vi "Decodificador_7seg_SubVI.vi"(1 "A":bool, 2 "B":bool, 3 "C":bool, 4 "D":bool) -> (0 "DISPLAY":T1)   [LabVIEW 2016]
doc: "Esta SubVI nos entrega a la salida un cluster que nos representa un dato binario en display de 7 segmentos."
panel:
  out "Segmento B":bool
  out "Segmento C":bool
  out "Segmento D":bool
  out "Segmento E":bool
  out "Segmento F":bool
  out "Segmento G":bool
  out "Segmento A":bool
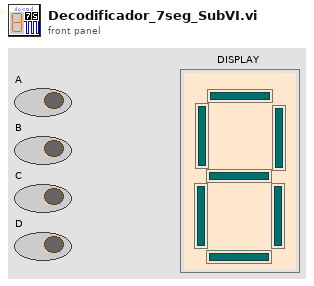
[diagram p1: front panel]
types:
  T1 = cluster{"SA":bool, "SB":bool, "SC":bool, "SD":bool, "SE":bool, "SF":bool, "SG":bool}
  T2 = cluster{bool, bool, bool, bool, bool, bool, bool}
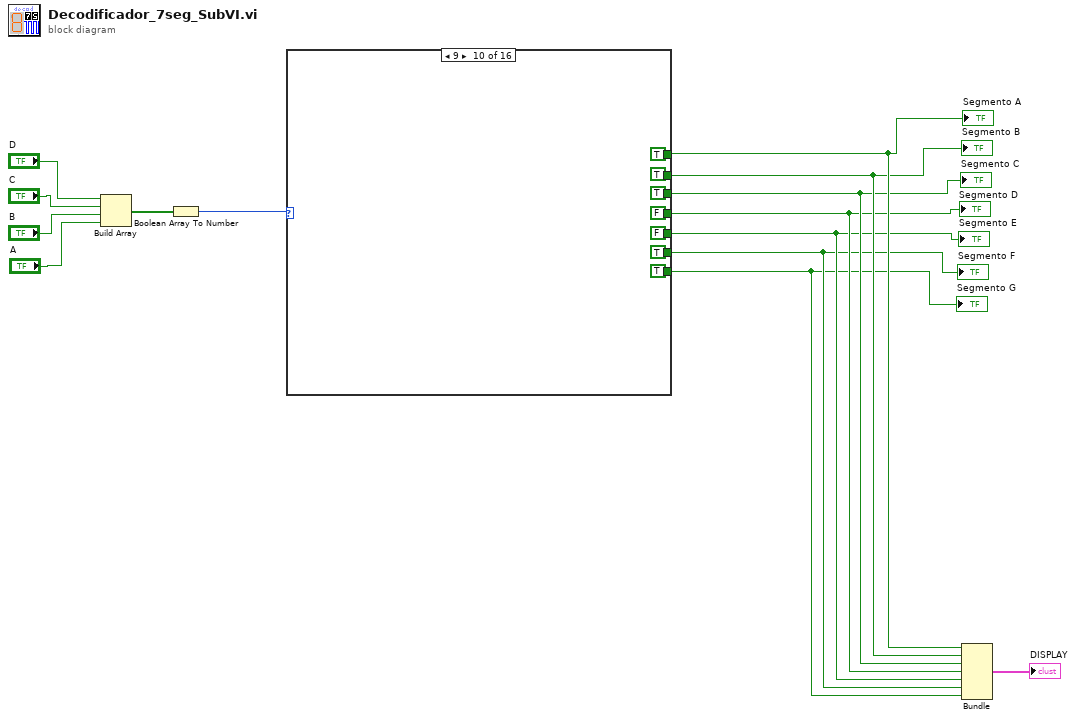
[diagram p0: block diagram]
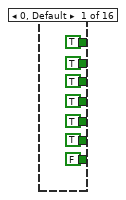
[diagram p2: hidden frame]
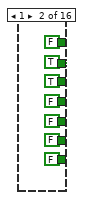
[diagram p3: hidden frame]
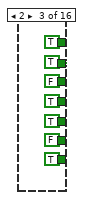
[diagram p4: hidden frame]
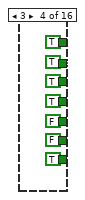
[diagram p5: hidden frame]
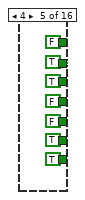
[diagram p6: hidden frame]
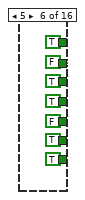
[diagram p7: hidden frame]
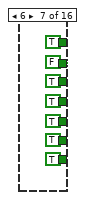
[diagram p8: hidden frame]
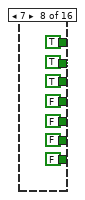
[diagram p9: hidden frame]
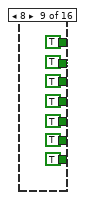
[diagram p10: hidden frame]
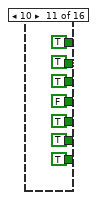
[diagram p11: hidden frame]
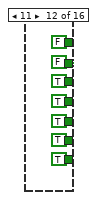
[diagram p12: hidden frame]
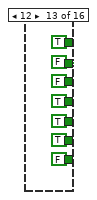
[diagram p13: hidden frame]
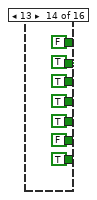
[diagram p14: hidden frame]
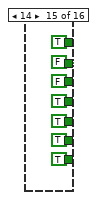
[diagram p15: hidden frame]
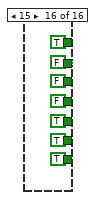
[diagram p16: hidden frame]
diagram:
  n1 = Build Array("D", "C", "B", "A") -> (w14:bool[])
  n2 = Boolean Array To Number(Boolean array=w14) -> (number=w9:u32)
  n3 = case shown="9" w9 {
    tunnel: [TRUE FALSE TRUE TRUE FALSE TRUE TRUE TRUE TRUE TRUE TRUE FALSE TRUE FALSE TRUE TRUE] -> w7
    tunnel: [TRUE TRUE TRUE TRUE TRUE FALSE FALSE TRUE TRUE TRUE TRUE FALSE FALSE TRUE FALSE FALSE] -> w6
    tunnel: [TRUE TRUE FALSE TRUE TRUE TRUE TRUE TRUE TRUE TRUE TRUE TRUE FALSE TRUE FALSE FALSE] -> w5
    tunnel: [TRUE FALSE TRUE TRUE FALSE TRUE TRUE FALSE TRUE FALSE FALSE TRUE TRUE TRUE TRUE FALSE] -> w4
    tunnel: [TRUE FALSE TRUE FALSE FALSE FALSE TRUE FALSE TRUE FALSE TRUE TRUE TRUE TRUE TRUE TRUE] -> w3
    tunnel: [TRUE FALSE FALSE FALSE TRUE TRUE TRUE FALSE TRUE TRUE TRUE TRUE TRUE FALSE TRUE TRUE] -> w2
    tunnel: [FALSE FALSE TRUE TRUE TRUE TRUE TRUE FALSE TRUE TRUE TRUE TRUE FALSE TRUE TRUE TRUE] -> w1
    frame 0, Default {
    }
    frame 1 {
    }
    frame 2 {
    }
    frame 3 {
    }
    frame 4 {
    }
    frame 5 {
    }
    frame 6 {
    }
    frame 7 {
    }
    frame 8 {
    }
    frame 9 {
    }
    frame 10 {
    }
    frame 11 {
    }
    frame 12 {
    }
    frame 13 {
    }
    frame 14 {
    }
    frame 15 {
    }
  }
  "Segmento A" <- w7
  "Segmento G" <- w1
  "Segmento F" <- w2
  "Segmento E" <- w3
  "Segmento D" <- w4
  "Segmento C" <- w5
  "Segmento B" <- w6
  n4 = Bundle(w7, w6, w5, w4, w3, w2, w1) -> (→"DISPLAY":T2)  [unwired: 1 in]
